vi "Gyro Align.vi"(6 "Reset Setpoint":bool, 8 "Current Gyro Val":dbl, 11 "Joystick Control":dbl) -> (1 "Output":dbl)   [LabVIEW 2014]
uses:
  <vilib>/addons/control/pid/pid.llb/PID (DBL).vi
  <vilib>/addons/control/pid/NI_PID_pid.lvlib
panel:
  out "Setpoint":dbl
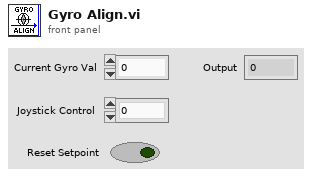
[diagram p1: front panel]
types:
  T1 = cluster{"proportional gain (Kc)":dbl, "integral time (Ti, min)":dbl, "derivative time (Td, min)":dbl}
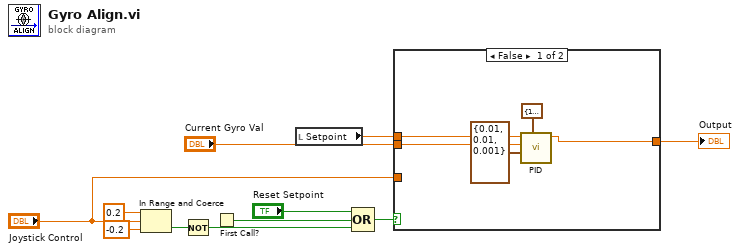
[diagram p0: block diagram]
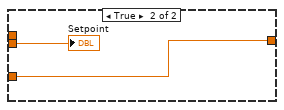
[diagram p2: hidden frame]
diagram:
  n1 = In Range and Coerce(upper limit=0.2, x="Joystick Control", lower limit=-0.2 ("y")) -> (In Range?=w8:bool)  [unwired: 1 out]
  n2 = Not(x=w8) -> (.not. x?=w1:bool)
  n3 = First Call?() -> (First Call?: T/F=w3:bool)
  n4 = local read "Setpoint"() -> (w7:dbl)
  n5 = Compound Arithmetic op=OR("Reset Setpoint", w3, w1) -> (w2:bool)
  n6 = case shown="False" w2 {
    tunnel: w7 -> [w14 _]
    tunnel: "Current Gyro Val" -> [w16 w18]
    tunnel: [w13 w17] -> w6
    tunnel: "Joystick Control" -> [_ w17]
    frame False {
      n7 = call-poly <vilib>:"PID.vi"("output range"=cluster{"output high":dbl, "output low":dbl} {"output high"=1.0, "output low"=-1.0}, "PID gains"=T1 {"proportional gain (Kc)"=0.01, "integral time (Ti, min)"=0.01, "derivative time (Td, min)"=0.001}, "process variable"=w16, "setpoint"=w14) -> ("output"=w13:dbl)  [unwired: 6 in, 1 out]
    }
    frame True {
      "Setpoint" <- w18
    }
  }
  "Output" <- w6
